vi "main.vi"() -> ()   [LabVIEW 2012]
uses:
  Controls/states.ctl
panel:
  out "Title":string="Price List Tool"
  in  "Check Marketing and\nService Items:":bool
  in  "OK Button":bool
  in  "Price List":path
  in  "Sample QB":path
  out "statusBar":string="Initialization....wait...."
  in  "Stop Button":bool
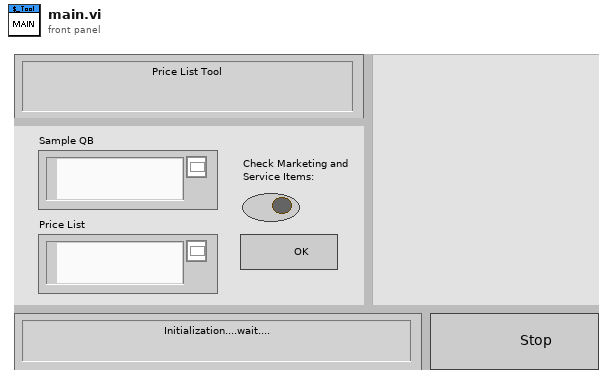
[diagram p1: front panel]
types:
  T1 = typedef "states.ctl" = enum16{"initiate", "waitEvent", "calculate", "stop"}
  T2 = cluster{"Excel._Application":refnum<k7>, "Workbooks":refnum<k7>, "Open":refnum<k7>, "Worksheets":refnum<k7>, "Excel._Worksheet":refnum<k7>}
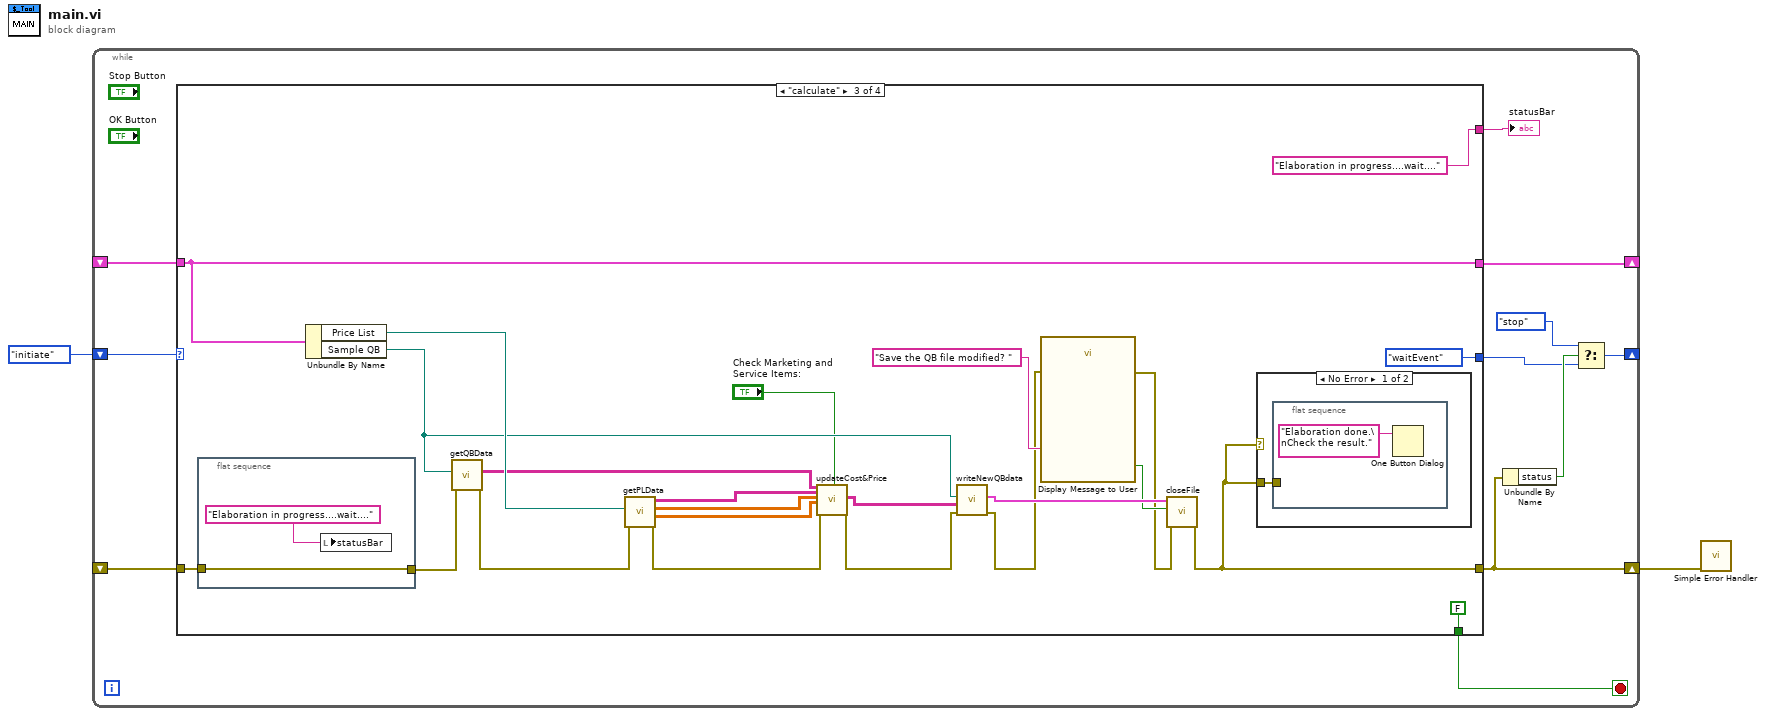
[diagram p0: block diagram]
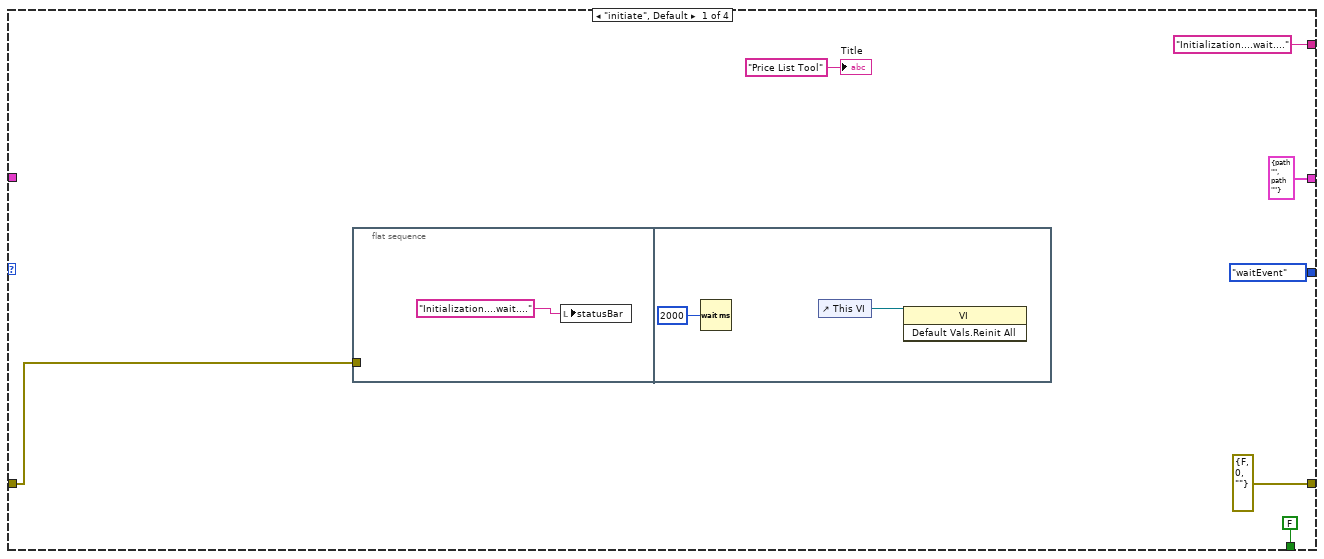
[diagram p2: hidden frame]
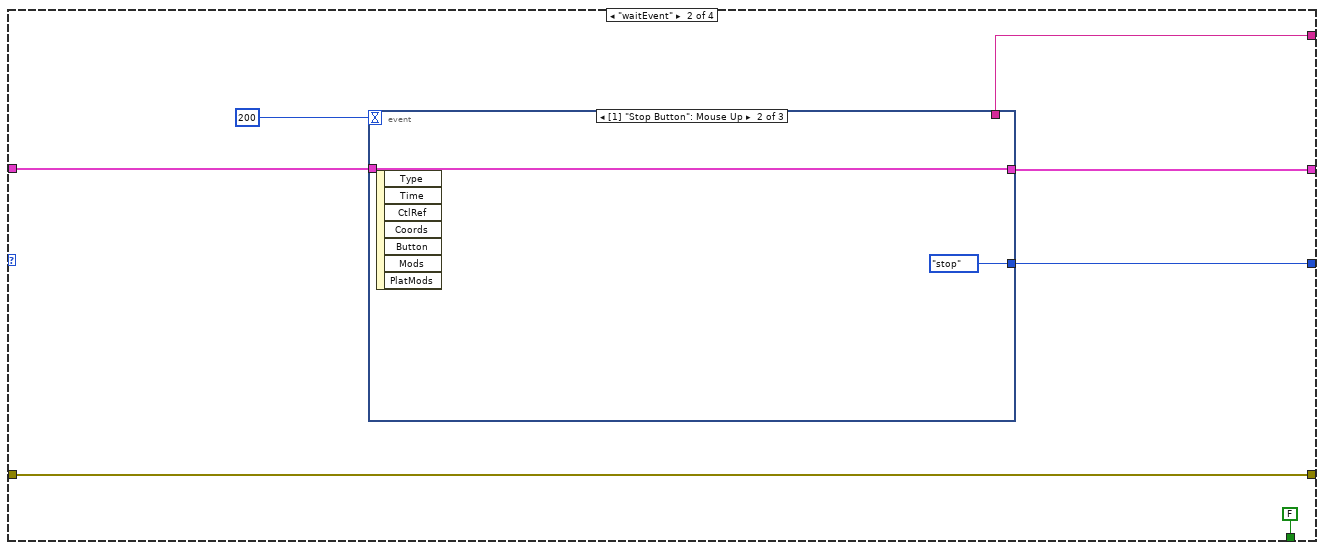
[diagram p3: hidden frame]
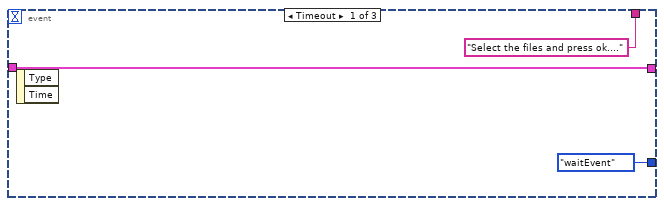
[diagram p4: hidden frame]
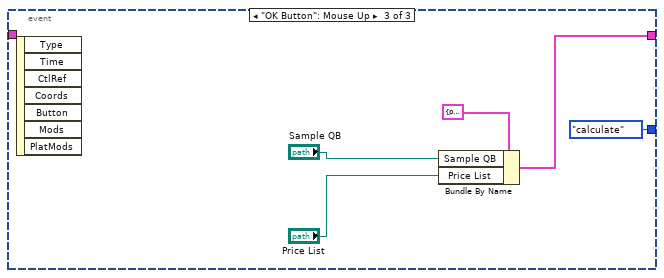
[diagram p5: hidden frame]
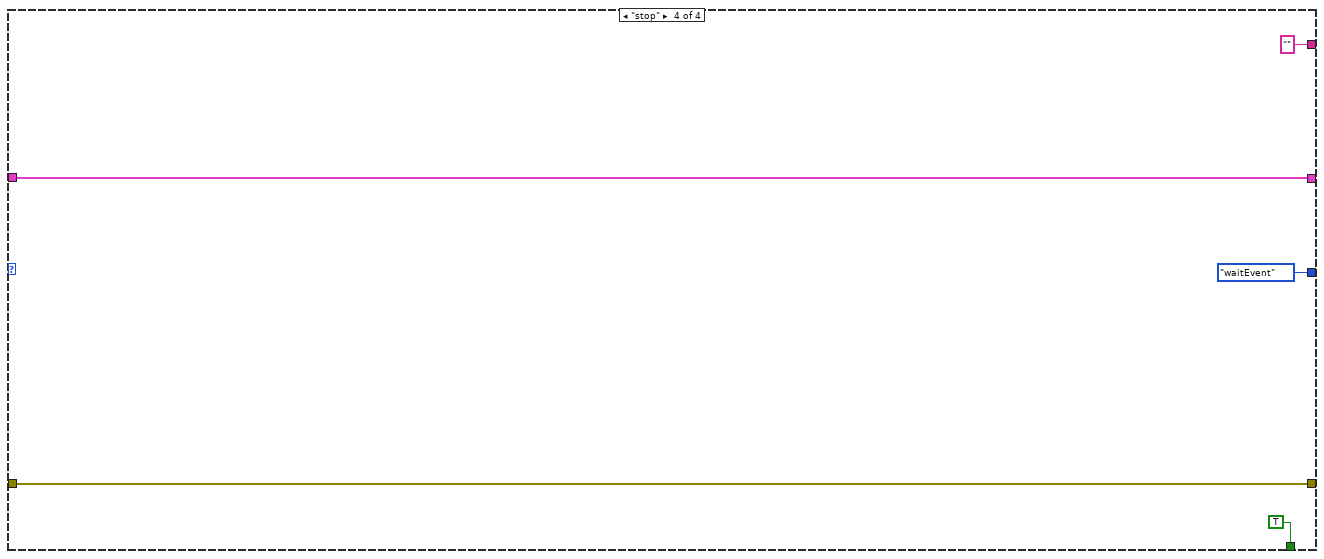
[diagram p7: hidden frame]
diagram:
  n1 = while {
    shift-right: [w5] -> _
    shift-left: states."initiate" ("state") -> [w13]
    shift-right: [w10] -> _
    shift-left: _ -> [w9]
    shift-right: [w7] -> w1
    shift-left: _ -> [w8]
    stop <- w11 stop-if-true
    n2 = case shown="\"calculate\"" w13 {
      tunnel: [states."waitEvent" ("state") w30 states."waitEvent" ("state") states."waitEvent" ("state")] -> w4
      tunnel: ["Initialization....wait...." ("Title") w25 "Elaboration in progress....wait...." ("Title") "" ("Title")] -> w12
      tunnel: [FALSE FALSE FALSE TRUE] -> w11
      tunnel: [cluster{"Sample QB":path, "Price List":path} {"Sample QB"=path "", "Price List"=path ""} w28 w58 w69] -> w10
      tunnel: w9 -> [_ w27 w58 w69]
      tunnel: [errorcluster {"status"=FALSE, "code"=0, "source"=""} ("error constant") w26 w41 w68] -> w7
      tunnel: w8 -> [w14 w26 w60 w68]
      frame "initiate", Default {
        n3 = flat-sequence {
          tunnel: w14 -> [_]
          frame #0 {
            n4 = local write "statusBar"("Initialization....wait...." ("Title")) -> ()
          }
          frame #1 {
            n5 = Wait (ms)(milliseconds to wait=u32 2000) -> ()  [unwired: 1 out]
            n6 = control-ref of="This VI"() -> (w22:refnum<vi>)
            n7 = invoke class="VI" method="Default Vals.Reinit All"(reference=w22) -> ()  [unwired: 2 in, 3 out]
          }
        }
        "Title" <- "Price List Tool" ("Title")
      }
      frame "waitEvent" {
        n8 = event shown="[1] \"Stop Button\": Mouse Up" {
          selector: _ -> [_ _ _]
          dyn-events: _ -> [_ _ _]
          timeout: 200 -> [_ _ _]
          tunnel: [states."waitEvent" ("state") states."stop" ("state") states."calculate" ("state")] -> w30
          tunnel: [w32 w34 w36] -> w28
          tunnel: w27 -> [w32 w34 _]
          tunnel: ["Select the files and press ok...." ("Title") _ _] -> w25
          event Timeout {
            n9 = event-data() -> ()  [unwired: 1 in, 2 out]
          }
          event "Stop Button": Mouse Up {
            n10 = event-data() -> ()  [unwired: 1 in, 7 out]
          }
          event "OK Button": Mouse Up {
            n11 = event-data() -> ()  [unwired: 1 in, 7 out]
            n12 = Bundle By Name(cluster=cluster{"Sample QB":path, "Price List":path} {"Sample QB"=path "", "Price List"=path ""}, "Sample QB"="Sample QB", "Price List"="Price List") -> (w36:cluster{"Sample QB":path, "Price List":path})
          }
        }
      }
      frame "calculate" {
        n13 = flat-sequence {
          tunnel: w60 -> [w67]
          tunnel: [w67] -> w59
          frame #0 {
            n14 = local write "statusBar"("Elaboration in progress....wait...." ("Title")) -> ()
          }
        }
        n15 = Unbundle By Name(w58) -> ("Price List"=w57:path, "Sample QB"=w48:path)
        n16 = call "getQBData.vi"("error in (no error)"=w59, "path"=w48) -> ("error out"=w61:errorcluster, "data"=w52:string[][])  [unwired: 8 in]
        n17 = call "getPLData.vi"("error in (no error)"=w61, "path"=w57) -> ("error out"=w56:errorcluster, "price"=w55:dbl[][], "cost"=w54:dbl[][], "data"=w53:string[][])  [unwired: 6 in]
        n18 = call "updateCost&Price.vi"("QBdata"=w52, "priceListData"=w53, "cost"=w54, "price"=w55, "error in (no error)"=w56, "marketing&&service"="Check Marketing and\nService Items:") -> ("newQBdata"=w50:string[][], "error out"=w49:errorcluster)  [unwired: 12 in]
        n19 = call "writeNewQBdata.vi"("error in (no error)"=w49, "newQBdata"=w50, "path"=w48) -> ("error out"=w44:errorcluster, "Refnum Cluster Out"=w47:T2)  [unwired: 7 in]
        n20 = call "Display Message to User"("error in (no error)"=w44, "Message"="Save the QB file modified? " ("message")) -> ("error out"=w43:errorcluster, "Save"=w45:bool)  [unwired: 8 in]
        n21 = call "closeFile.vi"("error in (no error)"=w43, "Save? (F)"=w45, "Refnum Cluster In"=w47) -> ("error out"=w41:errorcluster)  [unwired: 8 in]
        n22 = case shown="No Error" w41 {
          tunnel: w41 -> [w64 _]
          frame No Error {
            n23 = flat-sequence {
              tunnel: w64 -> [_]
              frame #0 {
                n24 = One Button Dialog(message="Elaboration done.\nCheck the result.") -> ()  [unwired: 1 in, 1 out]
              }
            }
          }
          frame Error {
          }
        }
      }
      frame "stop" {
      }
    }
    "statusBar" <- w12
    n25 = Unbundle By Name(w7) -> ("status"=w6:bool)
    n26 = Select(t=states."stop" ("f"), s=w6, f=w4) -> (s? t:f=w5:T1)
  }
  n27 = call <vilib>:"Simple Error Handler.vi"("error in (no error)"=w1) -> ()  [unwired: 4 in, 5 out]
